vi "PathController.vi"(7 "PID gains":T1={"proportional gain (Kc)"=1.0, "integral time (Ti, min)"=0.01, "derivative time (Td, min)"=0.0} {"derivative time (Td, min)" format="%.3f"; "integral time (Ti, min)" format="%.3f"; "proportional gain (Kc)" format="%.3f"}, 8 "reinitialize? (F)":bool, 9 "ThetaError":dbl, 10 "AheadLateralError":dbl, 11 "CurrentLateralError":dbl) -> (3 "Steering Voltage":dbl)   [LabVIEW 2013]
uses:
  <vilib>/addons/control/pid/pid.llb/PID (DBL).vi
  <vilib>/express/express arith-compare/Formula/XNode/ExpressFormulaBlockNode.xnode
  <vilib>/addons/control/pid/NI_PID_pid.lvlib
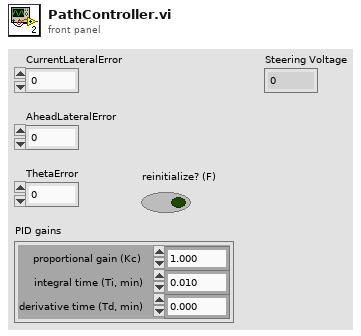
[diagram p1: front panel]
types:
  T1 = cluster{"proportional gain (Kc)":dbl, "integral time (Ti, min)":dbl, "derivative time (Td, min)":dbl}
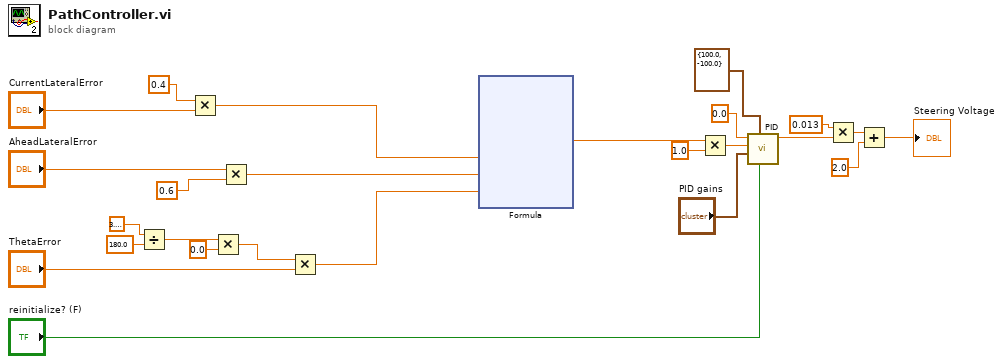
[diagram p0: block diagram]
diagram:
  n1 = Divide(x=3.141592653589793, y=180.0) -> (x/y=w15:dbl)
  n2 = Multiply(x=0.4 ("y"), y="CurrentLateralError") -> (x*y=w5:dbl)
  n3 = Multiply(x=w15, y=0.0) -> (x*y=w1:dbl)
  n4 = Multiply(x="AheadLateralError", y=0.6) -> (x*y=w4:dbl)
  n5 = Multiply(x=w1, y="ThetaError") -> (x*y=w3:dbl)
  n6 = xnode ("Formula")("X1"=w5, "X2"=w4, "X3"=w3) -> ("Result"=w18:dbl)  [unwired: 1 in, 1 out]
  n7 = Multiply(x=w18, y=1.0) -> (x*y=w10:dbl)
  n8 = call-poly <vilib>:"PID.vi"("reinitialize? (F)"="reinitialize? (F)", "output range"=cluster{"output high":dbl, "output low":dbl} {"output high"=100.0, "output low"=-100.0}, "PID gains"="PID gains", "process variable"=w10, "setpoint"=0.0) -> ("output"=w14:dbl)  [unwired: 5 in, 1 out]
  n9 = Multiply(x=0.013, y=w14) -> (x*y=w7:dbl)
  n10 = Add(x=w7, y=2.0) -> (x+y=→"Steering Voltage":dbl)
